vi "SendMultiPacket.vi"(8 "error in (no error)":errorcluster, 9 "PIDIn":u8, 10 "Packets In":T1[](array[typedef]), 11 "VISA resource name":refnum<visa-resource-name>) -> (0 "error out":errorcluster, 1 "PIDOut":u8, 2 "ReceivedBytes":T1[](array[typedef]), 3 "VISA resource name out":refnum<visa-resource-name>)   [LabVIEW 2009]
uses:
  Packet.ctl
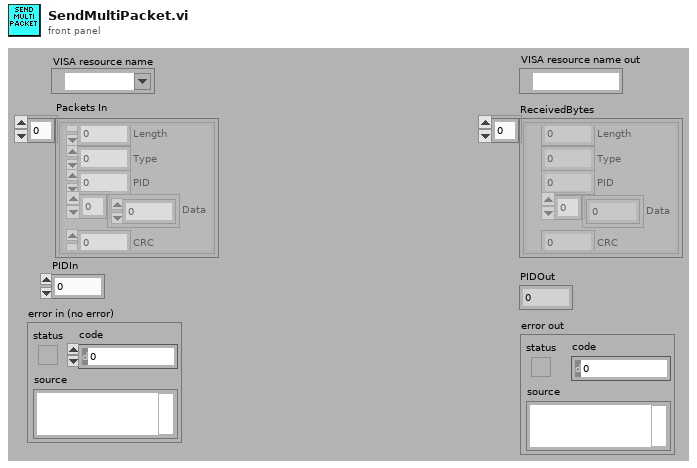
[diagram p1: front panel]
types:
  T1 = typedef "Packet.ctl" = cluster{"Length":u8, "Type":u8, "PID":u8, "Data":u8[], "CRC":u8}
  T2 = cluster{"Frame Byte":u8, "EscapeByte":u8, "XOR Byte":u8}
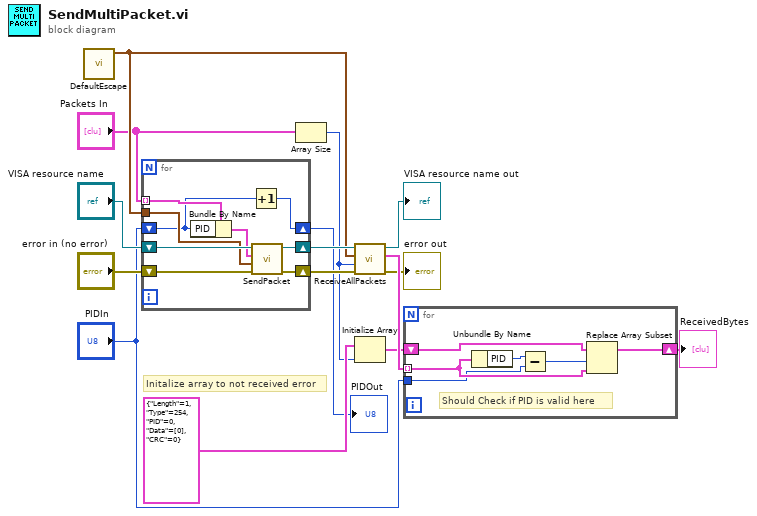
[diagram p0: block diagram]
diagram:
  # "Initalize array to not received error"
  n1 = call "DefaultEscape.vi"() -> ("EscapePattern"=w11:T2)  [unwired: 11 in]
  n2 = for {
    tunnel: "Packets In" -> [w19] mode=indexing
    shift-right: [w20] -> w12
    shift-left: "VISA resource name" -> [w24]
    shift-right: [w21] -> w10
    shift-left: "error in (no error)" -> [w23]
    tunnel: w11 -> [w22]
    shift-right: [w17] -> w2
    shift-left: "PIDIn" -> [w16]
    n3 = Bundle By Name(cluster=w19, "PID"=w16) -> (w18:T1)
    n4 = Increment(x=w16) -> (x+1=w17:u8)
    n5 = call "SendPacket.vi"("error in (no error)"=w23, "EscapePattern"=w22, "Transmit"=w18, "VISA resource name"=w24) -> ("error out"=w21:errorcluster, "VISA resource name out"=w20:refnum<visa-resource-name>)  [unwired: 6 in]
  }
  "PIDOut" <- w2
  n6 = Array Size(array="Packets In") -> (size(s)=w1:i32)
  n7 = call "ReceiveAllPackets.vi"("error in (no error)"=w10, "ExpectedPacketCount"=w1, "EscapePattern"=w11, "VISA resource name"=w12) -> ("error out"=→"error out":errorcluster, "ReceivedBytes"=w7:T1[], "VISA resource name out"=→"VISA resource name out":refnum<visa-resource-name>)  [unwired: 5 in]
  n8 = Initialize Array(T1 {"Length"=1, "Type"=254, "PID"=0, "Data"=[0], "CRC"=0} ("Packet"), w1) -> (w6:T1[])
  n9 = for {
    tunnel: w7 -> [w29] mode=indexing
    shift-right: [w30] -> w5
    shift-left: w6 -> [w28]
    tunnel: "PIDIn" -> [w25]
    # "Should Check if PID is valid here"
    n10 = Unbundle By Name(w29) -> ("PID"=w27:u8)
    n11 = Subtract(x=w27, y=w25) -> (x-y=w26:u8)
    n12 = Replace Array Subset(array=w28, new element=w29, index=w26) -> (w30:T1[])
  }
  "ReceivedBytes" <- w5
